vi "CLSUIP_SetNmdUnbundlerElement.vi"(8 "error in (no error)":errorcluster, 10 "Element Names":string[](array[string]), 11 "NmdUnbundler Ref":refnum<vi>) -> (0 "error out":errorcluster, 3 "NmdUnbundler Ref out":refnum<vi>)   [LabVIEW 2021, in "MemberVICreation.lvlib"]
uses:
  <resource>/Framework/Providers/LVClassLibrary/NewAccessors/MemberVICreation.lvlib
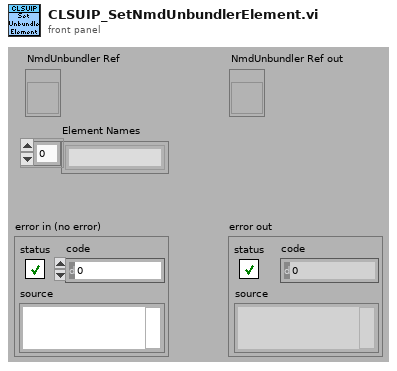
[diagram p1: front panel]
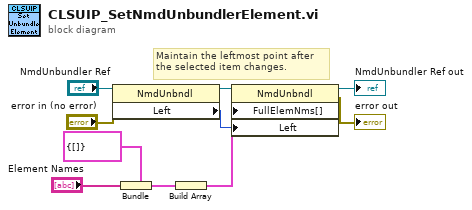
[diagram p0: block diagram]
diagram:
  # "Maintain the leftmost point after\nthe selected item changes."
  n1 = property class="NmdUnbndl"(reference="NmdUnbundler Ref", error in="error in (no error)") -> (reference out=w8:refnum<vi>, "Left"=w5:i32)  [unwired: 1 out]
  n2 = Bundle(cluster=cluster{string[]} {[]}, "Element Names") -> (w2:cluster{string[]})
  n3 = Build Array(w2) -> (w1:cluster{string[]}[])
  n4 = property class="NmdUnbndl"(reference=w8, "FullElemNms[]"=w1, "Left"=w5) -> (reference out=→"NmdUnbundler Ref out":refnum<vi>, error out=→"error out":errorcluster)  [unwired: 1 in]
